vi "libera_get.vi"(0 "handleConnection":T7, 1 "cuname":string, 2 "Enable ADC CW":bool, 3 "Enable DD":bool, 4 "sched (ms)":i32=100, 5 "cmd":string="status", 6 "Enable AVG":bool, 7 "args":string, 8 "timeout (10000)":i32=10000, 9 "Enable SA":bool, 10 "Enable ADC SP":bool, 14 "cmd submission mode":enum16{"stack", "kill previous"}(ring), 15 "prio":i32=50) -> (11 "timestamp":u64, 12 "AVG":cluster{"AVG":i32}[](array[cluster]), 13 "SA":T3(array[cluster]), 16 "DD":T4(array[cluster]), 17 "acquisitions":u64, 18 "ADC_SP":T1(array[cluster]), 19 "ADC_CW":T2(array[cluster]), 20 "dev_error":bool, 21 "dev_state":T5, 22 "STATUS":string, 23 "libera_error":i32, 24 "nok":i32, 25 "mode":i32, 27 "samples":i32)   [LabVIEW 2014]
uses:
  <vilib>/httpClient/ClientHandle.ctl
  chaos-common-crest/LabVIEW/LV14/chaosui-crest/VIs/ChaosDevState.ctl
  chaos-common-crest/LabVIEW/LV14/chaosui-crest/chaosui-crest.lvlib
  <vilib>/httpClient/LabVIEWHTTPClient.lvlib
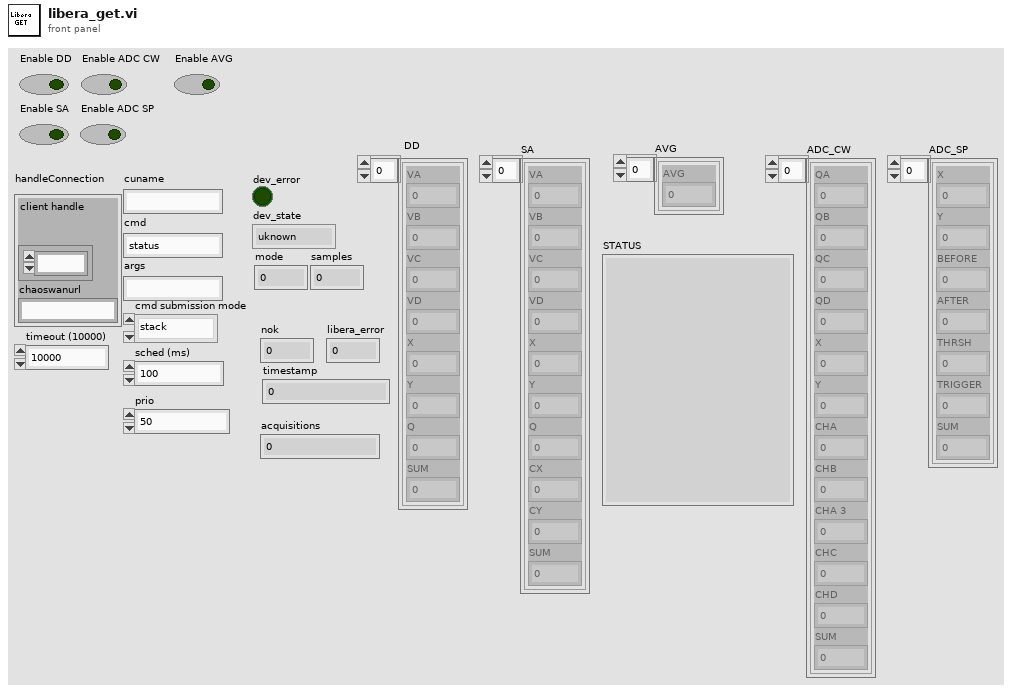
[diagram p1: front panel]
types:
  T1 = cluster{"X":i32, "Y":i32, "BEFORE":i32, "AFTER":i32, "THRSH":i32, "TRIGGER":i32, "SUM":i32}[]
  T2 = cluster{"QA":i32, "QB":i32, "QC":i32, "QD":i32, "X":i32, "Y":i32, "CHA":i32, "CHB":i32, "CHA 3":i32, "CHC":i32, "CHD":i32, "SUM":i32}[]
  T3 = cluster{"VA":i32, "VB":i32, "VC":i32, "VD":i32, "X":i32, "Y ":i32, "Q":i32, "CX":i32, "CY":i32, "SUM":i32}[]
  T4 = cluster{"VA":i32, "VB":i32, "VC":i32, "VD":i32, "X":i32, "Y ":i32, "Q":i32, "SUM":i32}[]
  T5 = typedef "ChaosDevState.ctl" = enum16{"uknown", "stop", "init", "deinit", "start"}
  T6 = typedef "LabVIEWHTTPClient.lvlib/ClientHandle.ctl" = refnum<k1>
  T7 = cluster{"client handle":T6, "chaoswanurl":string}
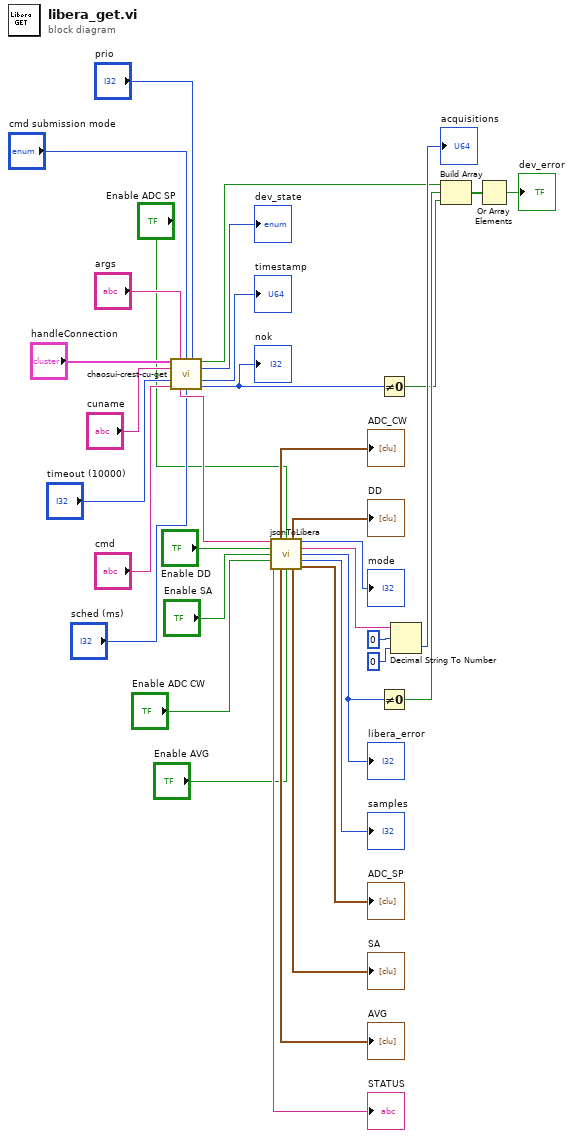
[diagram p0: block diagram]
diagram:
  n1 = call "chaosui-crest-cu-get.vi"("handleConnection"="handleConnection", "args"="args", "cmd submission mode"="cmd submission mode", "prio"="prio", "cuname"="cuname", "timeout (10000)"="timeout (10000)", "cmd"="cmd", "sched (ms)"="sched (ms)") -> ("dev_error"=w4:bool, "dev_state"=→"dev_state":T5, "timestamp"=→"timestamp":u64, "output out"=w29:string, "nok"=w5:i32)  [unwired: 3 in]
  "nok" <- w5
  n2 = call "jsonToLibera.vi"("json"=w29, "Enable ADC SP"="Enable ADC SP", "Enable DD"="Enable DD", "Enable SA"="Enable SA", "Enable ADC CW"="Enable ADC CW", "Enable AVG"="Enable AVG") -> ("ADC_CW"=→"ADC_CW":T2, "DD"=→"DD":T4, "mode"=→"mode":i32, "acquisitions"=w25:string, "libera_error"=w6:i32, "samples"=→"samples":i32, "STATUS"=→"STATUS":string, "AVG"=→"AVG":cluster{"AVG":i32}[], "SA"=→"SA":T3, "ADC_SP"=→"ADC_SP":T1)
  "libera_error" <- w6
  n3 = Not Equal To 0?(x=w5) -> (x != 0?=w1:bool)
  n4 = Not Equal To 0?(x=w6) -> (x != 0?=w2:bool)
  n5 = Decimal String To Number(string=w25, offset=0, default (0L)=u64 0 ("default (0 I32)")) -> (number=→"acquisitions":u64)  [unwired: 1 out]
  n6 = Build Array(w4, w2, w1) -> (w3:bool[])
  n7 = Or Array Elements(Boolean array=w3) -> (logical OR=→"dev_error":bool)
